vi "Get Selected Project Reference.vi"(8 "error in":errorcluster, 11 "Selected Project Name":string) -> (0 "error out":errorcluster, 2 "Project Refnum":refnum<vi>, 3 "Was Project Found?":bool)   [LabVIEW 2022 SP3]
doc: "<add documentation here>"
panel:
  # "Development\nControls or indicators that are useful for development or testing, but which are not outputs of the VI."
  # "Input\nInputs to the VI"
  # "Output\nOutputs of the VI"
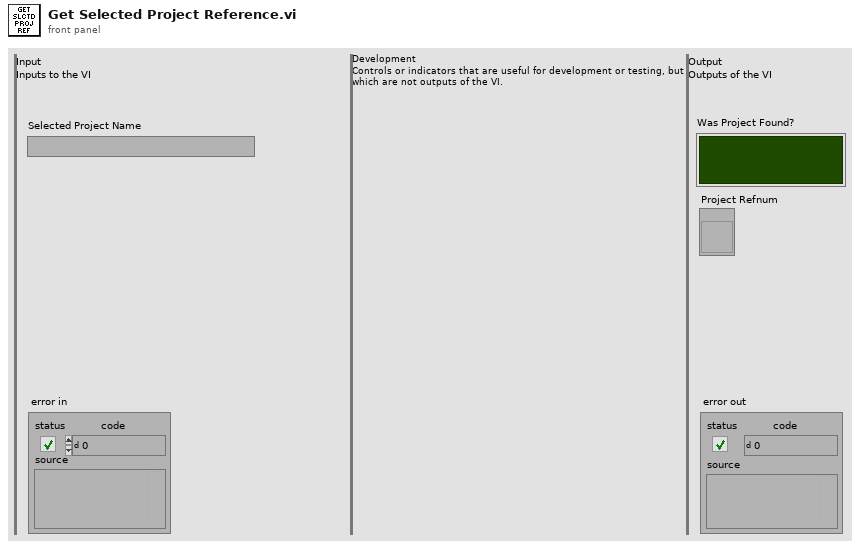
[diagram p1: front panel]
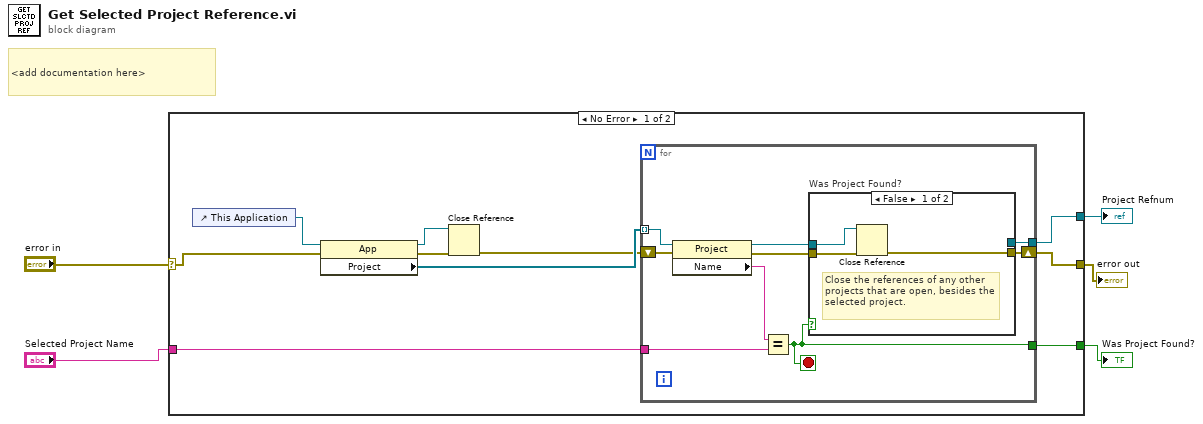
[diagram p0: block diagram]
diagram:
  # "<add documentation here>"
  n1 = case shown="No Error" "error in" {
    selector: "error in" -> [w8 w30]
    tunnel: "Selected Project Name" -> [w10 _]
    tunnel: [w9 _] -> w4
    tunnel: [w7 w30] -> w2
    tunnel: [w6 _] -> w1
    frame No Error {
      n2 = control-ref of="This Application"() -> (w14:refnum<vi>)
      n3 = property class="App"(reference=w14, error in=w8) -> (reference out=w11:refnum<vi>, error out=w15:errorcluster, "Project"=w13:refnum<vi>[])
      n4 = Close Reference(reference=w11, error in (no error)=w15) -> (error out=w12:errorcluster)
      n5 = for {
        shift-right: [w19] -> w7
        shift-left: w12 -> [w24]
        tunnel: w13 -> [w22] mode=indexing
        tunnel: w10 -> [w20]
        tunnel: [w17] -> w6
        tunnel: [w16] -> w9
        stop <- w17 stop-if-true
        n6 = property class="Project"(reference=w22, error in=w24) -> (reference out=w18:refnum<vi>, error out=w23:errorcluster, "Name"=w21:string)
        n7 = Equal?(x=w21, y=w20) -> (x = y?=w17:bool)
        n8 = case "Was Project Found?" shown="False" w17 {
          tunnel: w23 -> [w27 w28]
          tunnel: [w26 w28] -> w19
          tunnel: w18 -> [w25 w29]
          tunnel: [_ w29] -> w16
          frame False {
            # "Close the references of any other projects that are open, besides the selected project."
            n9 = Close Reference(reference=w25, error in (no error)=w27) -> (error out=w26:errorcluster)
          }
          frame True {
          }
        }
      }
    }
    frame Error {
    }
  }
  "Project Refnum" <- w4
  "error out" <- w2
  "Was Project Found?" <- w1
